vi "generate_ID_sequence.vi"(7 "stimulus":string(combo), 8 "user sequence":bool, 9 "randomize":bool, 10 "sequence IDs with spaces":string, 11 "blank time (s)":string) -> (3 "ID sequence":string)   [LabVIEW 2010, in "StimulatorAK101022TCP.lvclass"]
uses:
  StimulatorAK101022TCP.lvclass
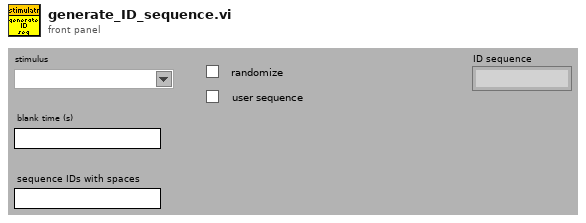
[diagram p1: front panel]
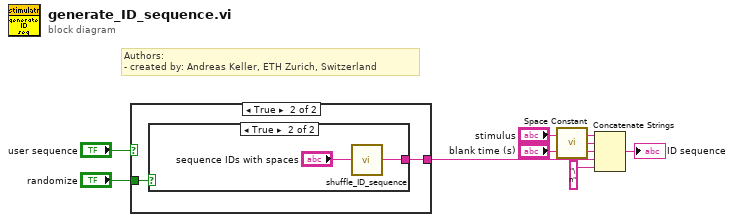
[diagram p0: block diagram]
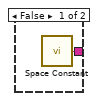
[diagram p2: hidden frame]
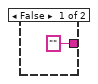
[diagram p3: hidden frame]
diagram:
  # "Authors: \n- created by: Andreas Keller, ETH Zurich, Switzerland"
  n1 = case shown="True" "user sequence" {
    tunnel: [w9 w10] -> w5
    tunnel: "randomize" -> [_ w11]
    frame False {
      n2 = call <vilib>:"Space Constant.vi"() -> ("String"=w9:string)
    }
    frame True {
      n3 = case shown="True" w11 {
        tunnel: ["" ("sequence IDs with spaces") w13] -> w10
        frame False {
        }
        frame True {
          n4 = call "shuffle_ID_sequence.vi"("sequence IDs with spaces"="sequence IDs with spaces") -> ("shuffled IDs"=w13:string)  [unwired: 10 in]
        }
      }
    }
  }
  n5 = call <vilib>:"Space Constant.vi"() -> ("String"=w3:string)
  n6 = Concatenate Strings("stimulus", w3, "blank time (s)", w5, "\n" ("string")) -> (→"ID sequence":string)
